vi "Eagle Scanner and Illumination Control.vi"() -> ()   [LabVIEW 2015]
uses:
  <vilib>/Utility/miscctls.llb/LVRectTypeDef.ctl
  <vilib>/userdefined/High Color/IMAQdx.ctl
  <vilib>/FPGAPlugInAG/cRIO-9030/niLvFpga_Open_cRIO-9030.vi
  <vilib>/rvi/interface/common/dynamic/niFpgaDynamicAddResources.vi
  <vilib>/Utility/error.llb/Error Cluster From Error Code.vi
  <vilib>/rvi/errors/niLvFpgaAdjustHostInterfaceError.vi
  <vilib>/rvi/interface/nirviOpenFPGA/nirviOpenFPGA.xnode
  FPGA Bitfiles/BELKINEAGLEGUI_FPGATarget_EagleFPGAScanner_juOkZGXIgM0.lvbitx
  <vilib>/rvi/interface/nirviReadWriteControl/nirviReadWriteControl.xnode
  <vilib>/rvi/interface/Simulation/niFpgaSimulationCallBeginRW.vi
  NiFpgaLv.dll
panel:
  out "Stopped":bool
  in  "Send":bool
  out "Y IND":fxp<+/-,20,5>
  out "X IND":fxp<+/-,20,5>
  in  "Scanner Y":dbl(slide)=1.5068493150684925 caption="Y Control" min=-10.0 max=10.0 step=1.0 scale=-10.0..10.0 scale format="%#.3g"
  in  "Scanner X":dbl(slide)=6.712328767123287 caption="X Control" min=-10.0 max=10.0 step=1.0 scale=-10.0..10.0 scale format="%#.3g"
  in  "Red Dots Ctrl":dbl(slide)=1.0 caption="Red Dots" max=10.0 step=1.0 scale=0.01..10.0 scale format="%#.3g"
  in  "V Range Ctrl":dbl(slide)=1.0 caption="V Range" max=10.0 step=1.0 scale=0.01..10.0 scale format="%#.3g"
  in  "LED Ctrl":dbl(slide)=1.0 caption="LED Ring" max=10.0 step=1.0 scale=0.01..10.0 scale format="%#.3g"
  in  "H Range Ctrl":dbl(slide)=1.0 caption="H Range" max=10.0 step=1.0 scale=0.01..10.0 scale format="%#.3g"
  in  "Aiming Ctrl":dbl(slide)=1.0 caption="Aiming" max=10.0 step=1.0 scale=0.01..10.0 scale format="%#.3g"
  out "ViewFinder Sign":picture
  out "Image":T1(plugin-control)
  in  "stop":bool
  # "EAGLE SYSTEM BASIC CONTROL"
  # "Scanner Control"
  # "Intensity Control"
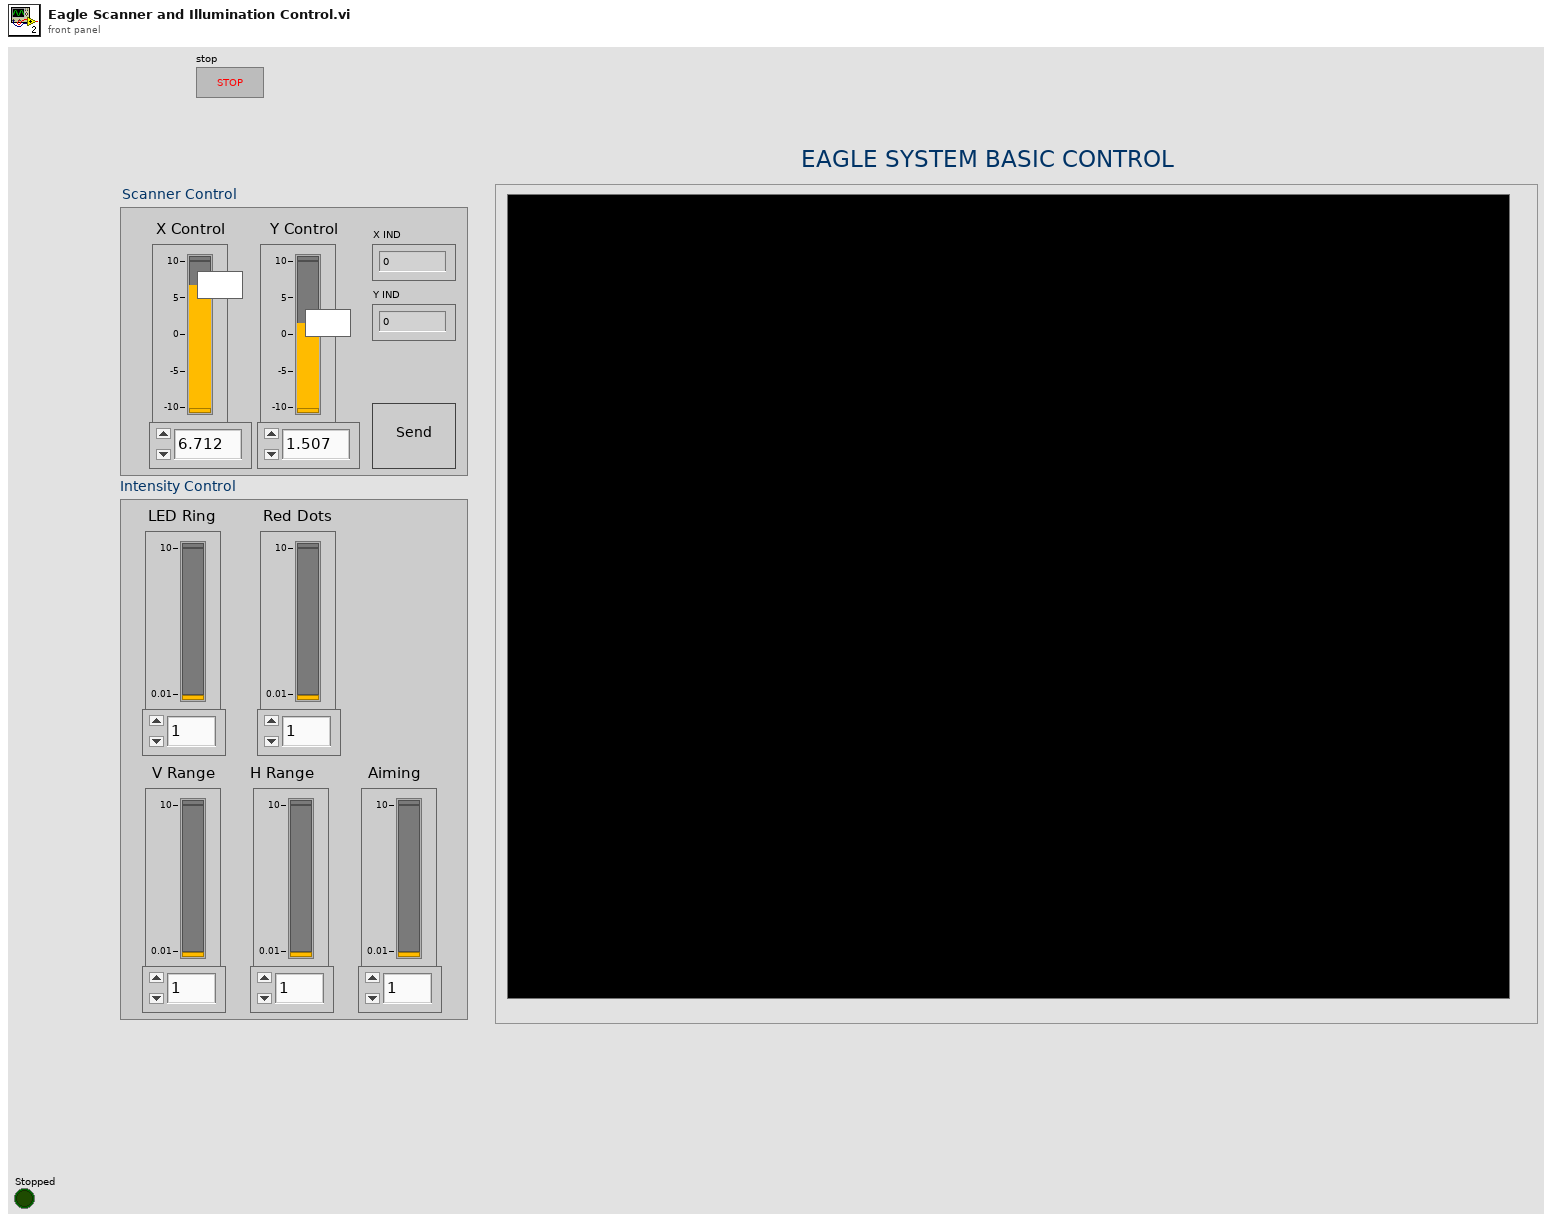
[diagram p1: front panel]
types:
  T1 = typedef "IMAQ Image.ctl" = refnum<image>
  T2 = typedef "LVRectTypeDef.ctl" = cluster{"Left":i16, "Top":i16, "Right":i16, "Bottom":i16}
  T3 = typedef "IMAQdx.ctl" = refnum<k21>
  T4 = typedef "Image Type" = u32
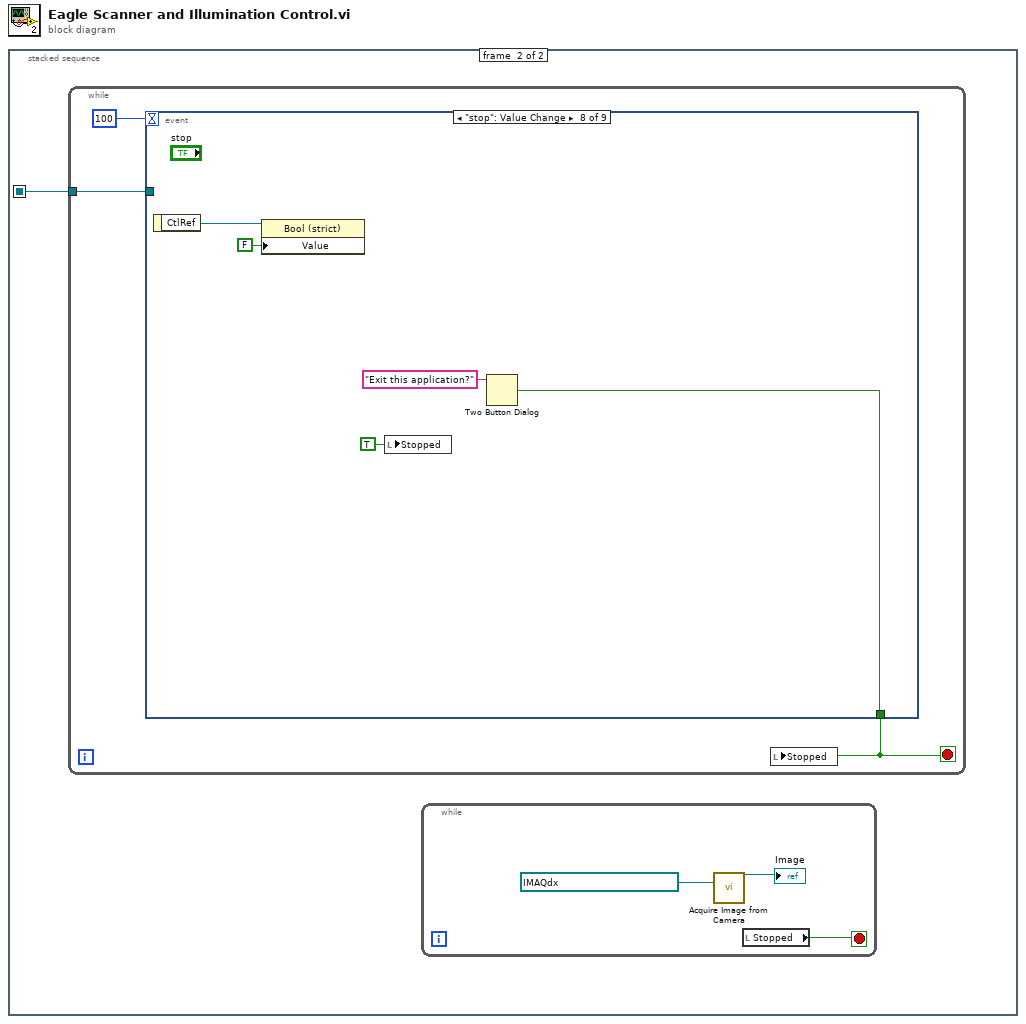
[diagram p0: block diagram]
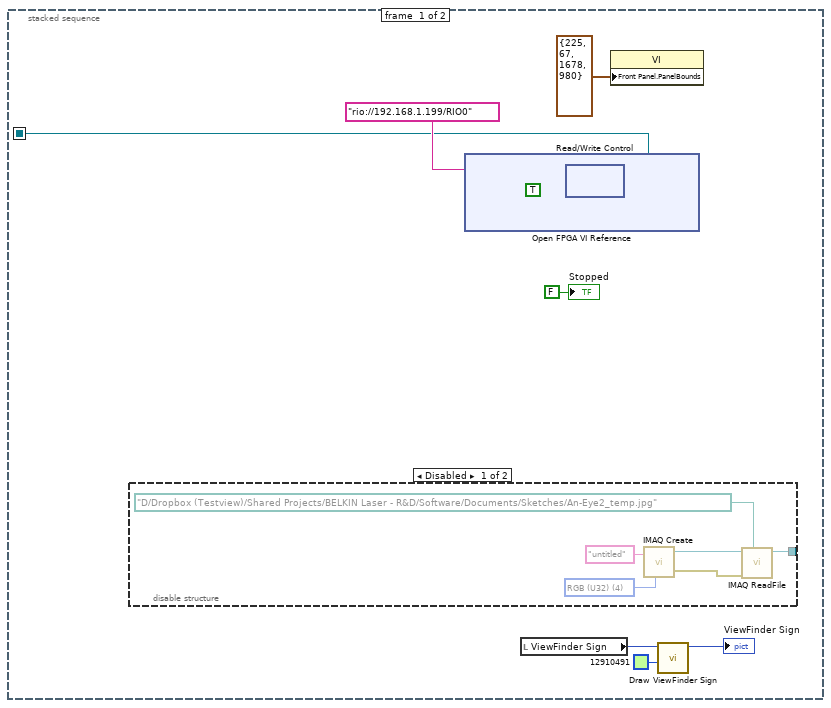
[diagram p2: hidden frame]
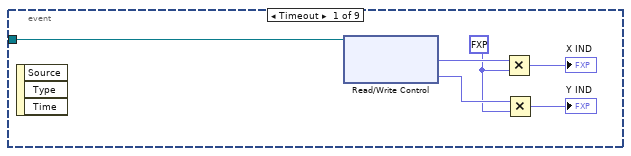
[diagram p4: hidden frame]
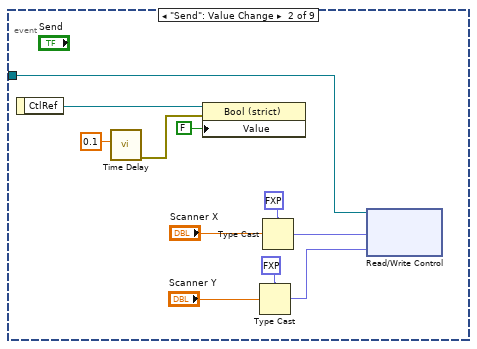
[diagram p5: hidden frame]
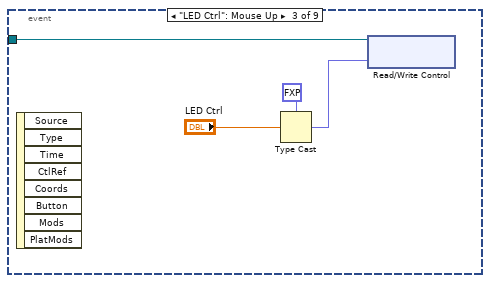
[diagram p6: hidden frame]
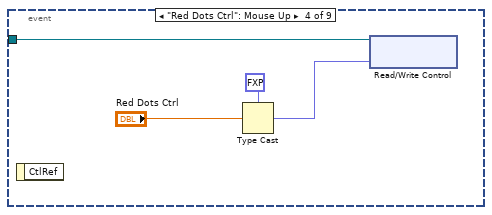
[diagram p7: hidden frame]
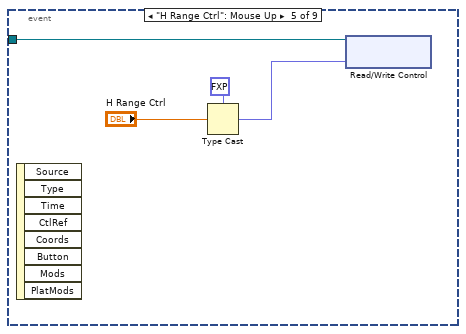
[diagram p8: hidden frame]
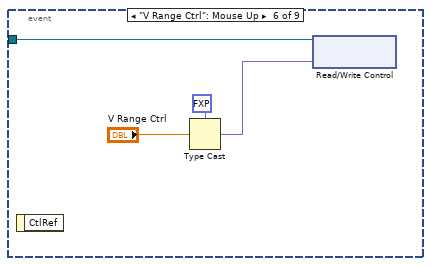
[diagram p9: hidden frame]
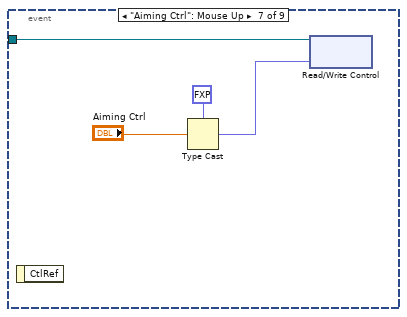
[diagram p10: hidden frame]
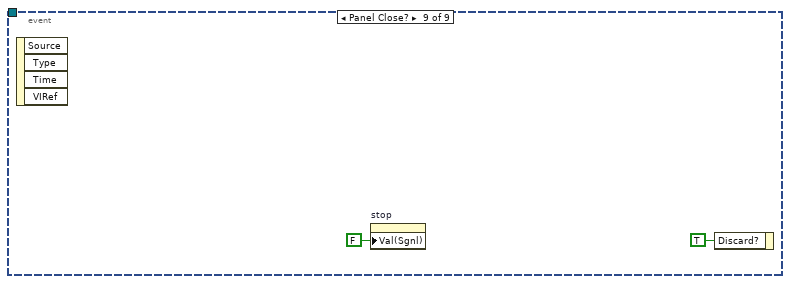
[diagram p11: hidden frame]
diagram:
  n1 = stacked-sequence {
    seq-local: [w2 _] -> [_ w16]
    frame #0 {
      n2 = disable-structure shown="Disabled" {
        disable-tunnel: [w10 _] -> _
        frame Disabled {
          w13 = T4 4 items=["Grayscale (U8)", "Grayscale (I16)", "Grayscale (SGL)", "Complex (CSG)", "RGB (U32)", "HSL (U32)", "RGB (U64)", "Grayscale (U16)"] ("Image Type")
          n3 = call "IMAQ Create"("Image Name"="untitled", "Image Type"=w13) -> ("New Image"=w12:T1, "error out"=w15:errorcluster)  [unwired: 3 in]
          n4 = call "IMAQ ReadFile"("File Path"=path "D:/Dropbox (Testview)/Shared Projects/BELKIN Laser - R&D/Software/Documents/Sketches/An-Eye2_temp.jpg", "error in (no error)"=w15, "Image"=w12) -> ("Image Out"=w10:T1)  [unwired: 4 in, 4 out]
        }
        frame Enabled {
        }
      }
      n5 = xnode "Open FPGA VI Reference"("resource name"=tag "rio://192.168.1.199/RIO0") -> ("FPGA VI Reference Out"=w4:refnum<k20>)  [unwired: 1 in, 1 out]
      n6 = local read "ViewFinder Sign"() -> (w5:picture)
      n7 = xnode "Read/Write Control"("FPGA VI Reference In"=w4, "Manual"=TRUE) -> ("FPGA VI Reference Out"=w2:refnum<k20>)  [unwired: 1 in, 1 out]
      n8 = property class="VI"("Front Panel.PanelBounds"=T2 {"Left"=225, "Top"=67, "Right"=1678, "Bottom"=980} ("Front Panel Window:Panel Bounds")) -> ()  [unwired: 2 in, 2 out]
      n9 = call "Draw ViewFinder Sign.vi"("Color"=u32 12910491, "2D Picture"=w5) -> ("2D Picture out"=→"ViewFinder Sign":picture)  [unwired: 9 in]
      "Stopped" <- FALSE ("Stopped")
    }
    frame #1 {
      n10 = while {
        tunnel: w16 -> [w22]
        stop <- w20 stop-if-true
        n11 = event shown="[7] \"stop\": Value Change" {
          selector: _ -> [_ _ _ _ _ _ _ _ _]
          dyn-events: _ -> [_ _ _ _ _ _ _ _ _]
          timeout: 100 -> [_ _ _ _ _ _ _ _ _]
          tunnel: [_ _ _ _ _ _ _ w61 _] -> w20
          tunnel: w22 -> [w28 w35 w43 w47 w51 w55 w59 _ _]
          event Timeout {
            w24 = fxp<+/-,20,5> 2.0 ("X IND")
            n12 = event-data() -> ()  [unwired: 1 in, 3 out]
            n13 = xnode "Read/Write Control"("FPGA VI Reference In"=w28) -> ("Manual X IND"=w27:fxp<+/-,20,5>, "Manual Y IND"=w25:fxp<+/-,20,5>)  [unwired: 1 in, 2 out]
            n14 = Multiply(x=w27, y=w24) -> (x*y=→"X IND":fxp<+/-,40,10>)
            n15 = Multiply(x=w25, y=w24) -> (x*y=→"Y IND":fxp<+/-,40,10>)
          }
          event "Send": Value Change {
            n16 = event-data() -> ("CtlRef"=w39:refnum<vi>)  [unwired: 1 in]
            n17 = call "Time Delay"("Delay Time (s)"=0.1) -> ("error out"=w37:errorcluster)  [unwired: 10 in]
            n18 = property class="Bool (strict)"(reference=w39, error in=w37, "Value"=FALSE) -> ()  [unwired: 2 out]
            n19 = Type Cast(type=fxp<+/-,20,5> 0.0 ("Manual VX"), x="Scanner Y") -> (*(type *) &x=w30:fxp<+/-,20,5>)
            n20 = Type Cast(type=fxp<+/-,20,5> 0.0 ("Manual VX"), x="Scanner X") -> (*(type *) &x=w34:fxp<+/-,20,5>)
            n21 = xnode "Read/Write Control"("FPGA VI Reference In"=w35, "Manual VX"=w34, "Manual VY"=w30) -> ()  [unwired: 1 in, 2 out]
          }
          event "LED Ctrl": Mouse Up {
            n22 = event-data() -> ()  [unwired: 1 in, 8 out]
            n23 = Type Cast(type=fxp<+,16,3> 0.0 ("LED Ring Ctrl"), x="LED Ctrl") -> (*(type *) &x=w41:fxp<+,16,3>)
            n24 = xnode "Read/Write Control"("FPGA VI Reference In"=w43, "LED Ring Ctrl"=w41) -> ()  [unwired: 1 in, 2 out]
          }
          event "Red Dots Ctrl": Mouse Up {
            n25 = event-data() -> ()  [unwired: 1 in, 1 out]
            n26 = Type Cast(type=fxp<+,16,3> 0.0 ("Red Dots Ctrl"), x="Red Dots Ctrl") -> (*(type *) &x=w44:fxp<+,16,3>)
            n27 = xnode "Read/Write Control"("FPGA VI Reference In"=w47, "Red Dots Ctrl"=w44) -> ()  [unwired: 1 in, 2 out]
          }
          event "H Range Ctrl": Mouse Up {
            n28 = event-data() -> ()  [unwired: 1 in, 8 out]
            n29 = Type Cast(type=fxp<+,16,3> 0.0 ("H Range Ctrl"), x="H Range Ctrl") -> (*(type *) &x=w48:fxp<+,16,3>)
            n30 = xnode "Read/Write Control"("FPGA VI Reference In"=w51, "H Range Ctrl"=w48) -> ()  [unwired: 1 in, 2 out]
          }
          event "V Range Ctrl": Mouse Up {
            n31 = event-data() -> ()  [unwired: 1 in, 1 out]
            n32 = Type Cast(type=fxp<+,16,3> 0.0 ("V Range Ctrl"), x="V Range Ctrl") -> (*(type *) &x=w52:fxp<+,16,3>)
            n33 = xnode "Read/Write Control"("FPGA VI Reference In"=w55, "V Range Ctrl"=w52) -> ()  [unwired: 1 in, 2 out]
          }
          event "Aiming Ctrl": Mouse Up {
            n34 = event-data() -> ()  [unwired: 1 in, 1 out]
            n35 = Type Cast(type=fxp<+,16,3> 0.0 ("Aim Ctrl"), x="Aiming Ctrl") -> (*(type *) &x=w56:fxp<+,16,3>)
            n36 = xnode "Read/Write Control"("FPGA VI Reference In"=w59, "Aim Ctrl"=w56) -> ()  [unwired: 1 in, 2 out]
          }
          event "stop": Value Change {
            n37 = event-data() -> ("CtlRef"=w64:refnum<vi>)  [unwired: 1 in]
            n38 = property class="Bool (strict)"(reference=w64, "Value"=FALSE) -> ()  [unwired: 1 in, 2 out]
            n39 = local write "Stopped"(TRUE ("Stopped")) -> ()
            n40 = Two Button Dialog(message="Exit this application?") -> (T button?=w61:bool)  [unwired: 2 in]
          }
          event Panel Close? {
            n41 = event-data() -> ()  [unwired: 1 in, 4 out]
            n42 = property on="stop" class="Bool (strict)"("Val(Sgnl)"=FALSE ("Value (Signaling)")) -> ()  [unwired: 2 in, 2 out]
            n43 = event-data("Discard?"=TRUE) -> ()  [unwired: 1 in, 1 out]
          }
        }
        n44 = local write "Stopped"(w20) -> ()
      }
      n45 = while {
        stop <- w18 stop-if-true
        n46 = call "Acquire Image from Camera.vi"("Session In"=T3 "rio:\\\\192.168.1.199\\cam0") -> ("Image Out"=→"Image":T1)  [unwired: 23 in, 3 out]
        n47 = local read "Stopped"() -> (w18:bool)
      }
    }
  }
